vi "Init Teller.vi"(10 "Teller Elements":T1 {"Time" format="%<%x %.3X>T"}) -> (2 "Teller":refnum<class "Teller.lvclass">)   [LabVIEW 2020, in "jettl.lvlib" / "Base Teller.lvlib"]
uses:
  Base Teller.lvlib
  Teller/Teller.lvclass
  Base Teller/Base Teller.lvclass
  Teller Elements.ctl
  jettl.lvlib
  Relation.ctl
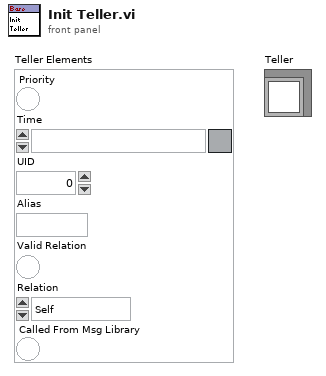
[diagram p1: front panel]
types:
  T1 = typedef "jettl.lvlib/Teller Elements.ctl" = cluster{"Priority":bool, "Time":timestamp, "UID":i32, "Alias":string, "Valid Relation":bool, "Relation":T2, "Called From Msg Library":bool}
  T2 = typedef "jettl.lvlib/Relation.ctl" = enum16{"Self", "Parent", "Child"}
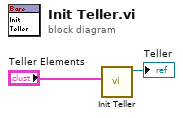
[diagram p0: block diagram]
diagram:
  n1 = call "Init Teller.vi"("Teller Elements"="Teller Elements") -> ("Base Teller out"=→"Teller":refnum<class "Base Teller.lvclass">)  [unwired: 10 in]
